vi "ArmNetworkingGlobal.vi"() -> ()   [LabVIEW 2023]
panel:
  out "LiftHighLimit":bool
  out "LiftFowardLimit":bool
  out "LiftFowardLimitL":bool
  out "LiftFowardLimitR":bool
  out "OnTarget":bool
  in  "LiftSensorPosition":dbl
  in  "LiftDemand":dbl
  in  "MotorOutput":dbl
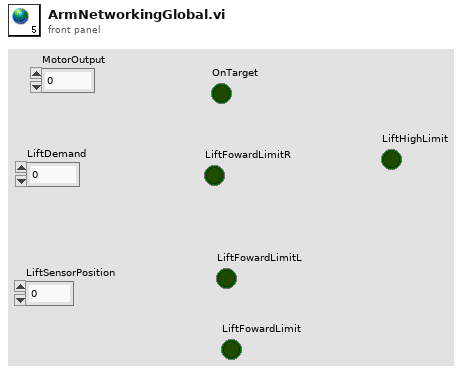
[diagram p1: front panel]
diagram:
